vi "OSC UDP Sender.vi"() -> ()   [LabVIEW 2013]
doc: "This example VI shows how to create Open Sound Control (OSC) messages and send them over UDP. This VI is intended to be run with the OSC UDP Receiver example VI."
uses:
  <vilib>/NIOSC/Create Float32 Argument.vi
  <vilib>/NIOSC/Create Double Argument.vi
  <vilib>/NIOSC/Create Boolean Argument.vi
  <vilib>/NIOSC/Create String Argument.vi
  <vilib>/NIOSC/Generate Error.vi
  <vilib>/NIOSC/Pad String.vi
  <vilib>/NIOSC/Check for Valid String Data.vi
  <vilib>/NIOSC/Multiple of 32.vi
  <vilib>/NIOSC/Create Message_Single Arg.vi
  <vilib>/NIOSC/Create Message_Multiple Args.vi
  <vilib>/NIOSC/NI_OSC.lvlib
panel:
  in  "/group4/data":T1
  in  "/group3/bool/*":bool
  in  "/group3/bool/c":bool
  in  "/group3/bool/b":bool
  in  "/group3/bool/a":bool
  in  "//float64//":dbl(slide) scale=-100.0..100.0
  in  "/group2/float64/num_a":dbl
  in  "/group2/float32/num_b":sgl
  in  "//float32//":sgl(slide) scale=-100.0..100.0
  in  "Yslide":sgl(slide) scale=-1.0..1.0
  in  "Zout":sgl(slide) scale=-20.0..10.0
  in  "Broadcast":bool
  in  "Remote Host":string="localhost"
  in  "Remote Port":u16=9000
  in  "Local Port":u16=7000
  in  "stop":bool
  # "Instructions:\n1. Open the receiver VI (OSC UDP Receiver.vi).\n2. Make sure the Remote Port in this VI and the Local Port in the receiver VI are the same.\n3. Run both VIs.\n4. Change the values of the controls on this VI to observe how OSC messages are created.  The indicators on the receiver VI should update."
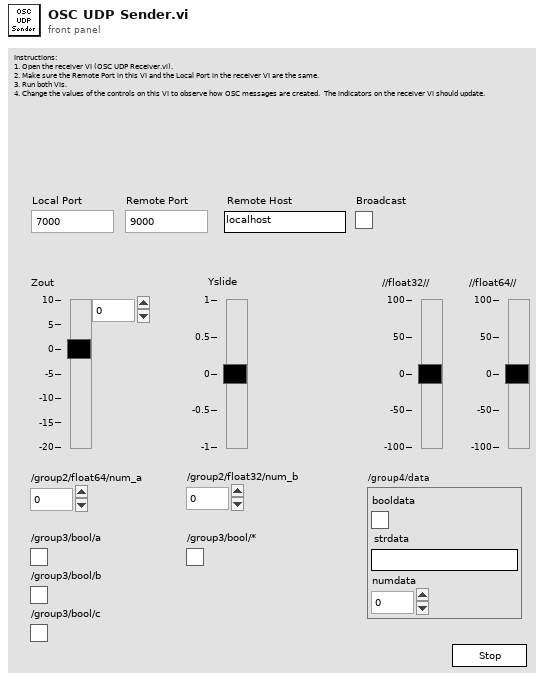
[diagram p1: front panel]
types:
  T1 = cluster{"booldata":bool, "strdata":string, "numdata":dbl}
  T2 = typedef "NI_OSC.lvlib/Argument.ctl" = cluster{"argument":string, "type tag":string}
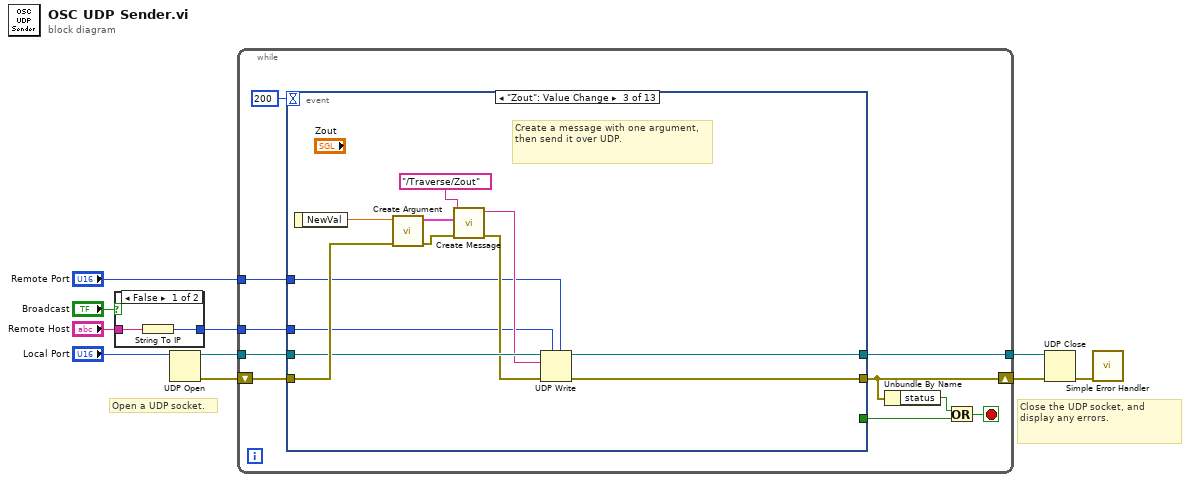
[diagram p0: block diagram]
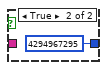
[diagram p2: hidden frame]
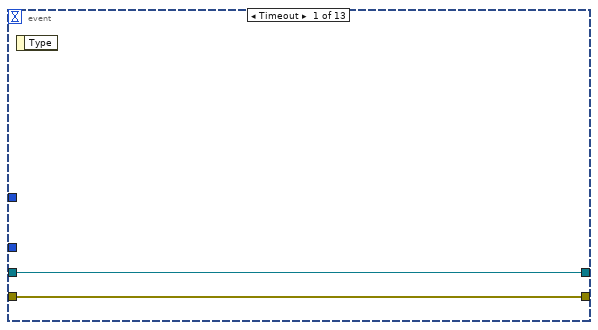
[diagram p3: hidden frame]
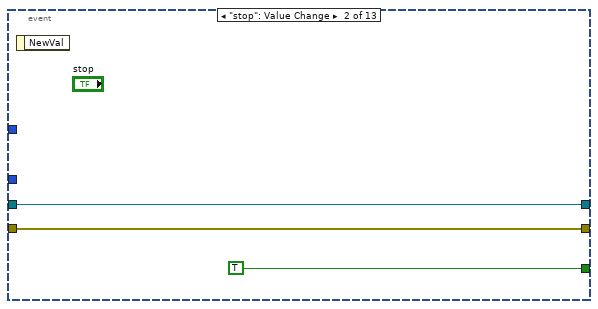
[diagram p4: hidden frame]
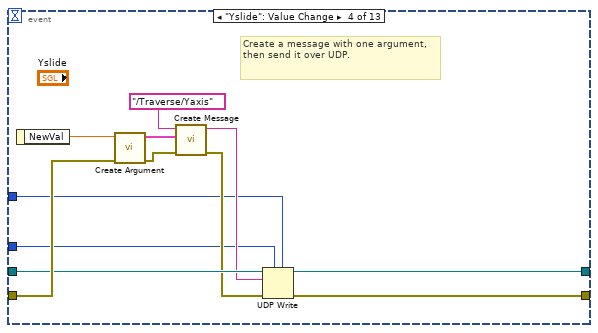
[diagram p5: hidden frame]
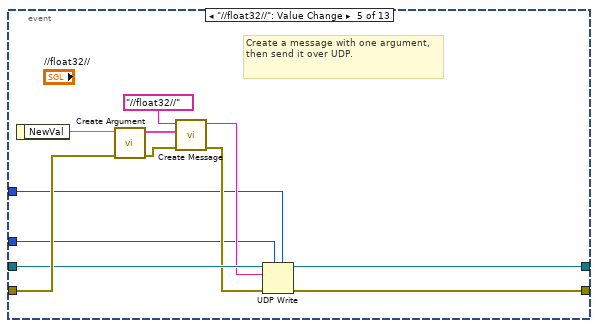
[diagram p6: hidden frame]
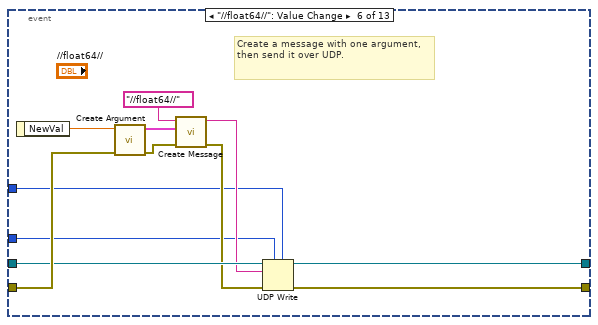
[diagram p7: hidden frame]
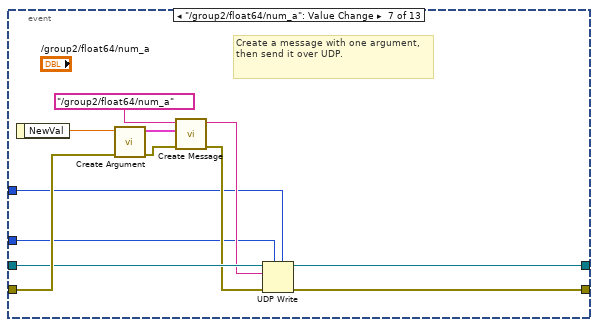
[diagram p8: hidden frame]
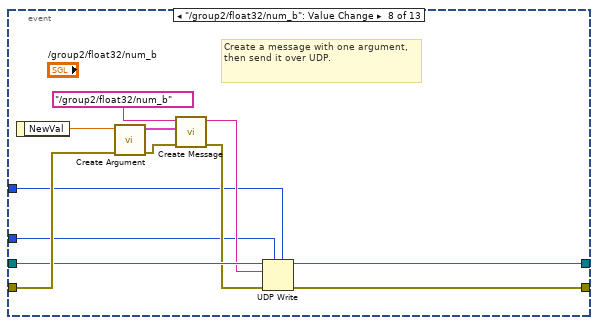
[diagram p9: hidden frame]
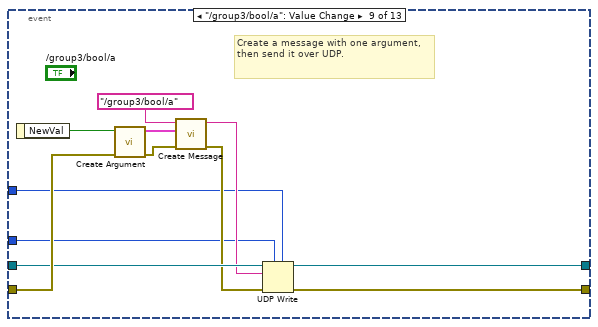
[diagram p10: hidden frame]
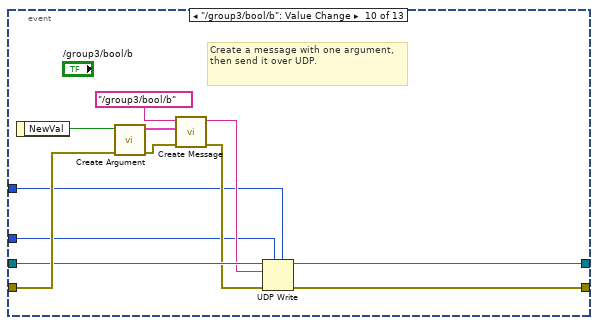
[diagram p11: hidden frame]
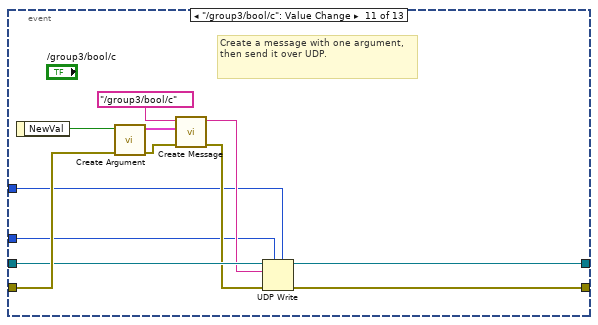
[diagram p12: hidden frame]
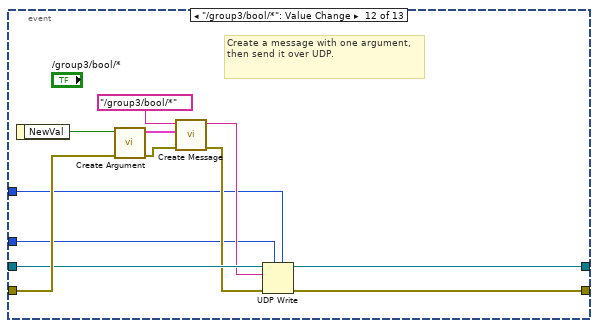
[diagram p13: hidden frame]
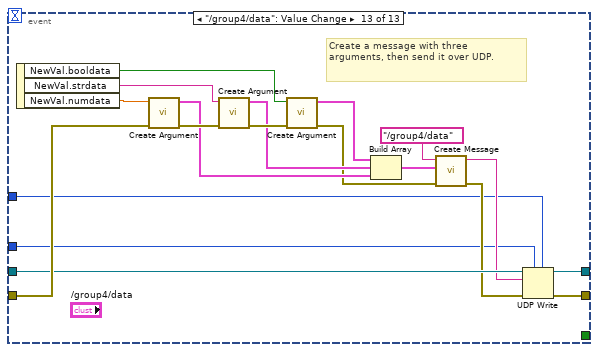
[diagram p14: hidden frame]
diagram:
  # "Close the UDP socket, and display any errors."
  # "Open a UDP socket."
  n1 = case shown="False" "Broadcast" {
    tunnel: "Remote Host" -> [w12 _]
    tunnel: [w11 u32 4294967295] -> w2
    frame False {
      n2 = String To IP(1:w12) -> (0:w11:u32)
    }
    frame True {
    }
  }
  n3 = UDP Open(11:"Local Port") -> (port=w9:refnum<k16>, 0:w8:errorcluster)  [unwired: 4 in, 1 out]
  n4 = while {
    tunnel: w9 -> [w22]
    shift-right: [w17] -> w5
    shift-left: w8 -> [w21]
    tunnel: "Remote Port" -> [w20]
    tunnel: [w19] -> w6
    tunnel: w2 -> [w18]
    stop <- w14 stop-if-true
    n5 = event shown="[2] \"Zout\": Value Change" {
      selector: _ -> [_ _ _ _ _ _ _ _ _ _ _ _ _]
      dyn-events: _ -> [_ _ _ _ _ _ _ _ _ _ _ _ _]
      timeout: 200 -> [_ _ _ _ _ _ _ _ _ _ _ _ _]
      tunnel: [_ TRUE _ _ _ _ _ _ _ _ _ _ _] -> w16
      tunnel: w22 -> [w25 w27 w36 w47 w59 w72 w84 w96 w108 w120 w132 w144 w165]
      tunnel: w21 -> [w24 w26 w37 w48 w60 w73 w85 w97 w109 w121 w133 w145 w166]
      tunnel: w20 -> [_ _ w32 w43 w55 w68 w80 w92 w104 w116 w128 w140 w161]
      tunnel: [w25 w27 w35 w46 w58 w71 w83 w95 w107 w119 w131 w143 w164] -> w19
      tunnel: [w24 w26 w30 w41 w53 w66 w78 w90 w102 w114 w126 w138 w159] -> w17
      tunnel: w18 -> [_ _ w31 w42 w54 w67 w79 w91 w103 w115 w127 w139 w160]
      event Timeout {
        n6 = event-data() -> ()  [unwired: 1 in, 1 out]
      }
      event "stop": Value Change {
        n7 = event-data() -> ()  [unwired: 1 in, 1 out]
      }
      event "Zout": Value Change {
        # "Create a message with one argument, then send it over UDP."
        n8 = event-data() -> ("NewVal"=w29:sgl)  [unwired: 1 in]
        n9 = call-poly <vilib>:"Create Argument.vi"("error in"=w37, "float32 data"=w29) -> ("error out"=w38:errorcluster, "float32 argument"=w40:T2)  [unwired: 8 in]
        n10 = call-poly <vilib>:"Create Message.vi"("error in"=w38, "argument"=w40, "address pattern"="/Traverse/Zout") -> ("error out"=w34:errorcluster, "message"=w33:string)  [unwired: 7 in]
        n11 = UDP Write(address=w31, port or service name=w32, connection ID=w36, data in=w33, 8:w34) -> (error out=w30:errorcluster, 3:w35:refnum<k16>)  [unwired: 1 in]
      }
      event "Yslide": Value Change {
        # "Create a message with one argument, then send it over UDP."
        n12 = event-data() -> ("NewVal"=w52:sgl)  [unwired: 1 in]
        n13 = call-poly <vilib>:"Create Argument.vi"("error in"=w48, "float32 data"=w52) -> ("error out"=w49:errorcluster, "float32 argument"=w51:T2)  [unwired: 8 in]
        n14 = call-poly <vilib>:"Create Message.vi"("error in"=w49, "argument"=w51, "address pattern"="/Traverse/Yaxis") -> ("error out"=w45:errorcluster, "message"=w44:string)  [unwired: 7 in]
        n15 = UDP Write(address=w42, port or service name=w43, connection ID=w47, data in=w44, 8:w45) -> (error out=w41:errorcluster, 3:w46:refnum<k16>)  [unwired: 1 in]
      }
      event "//float32//": Value Change {
        # "Create a message with one argument, then send it over UDP."
        n16 = event-data() -> ("NewVal"=w64:sgl)  [unwired: 1 in]
        n17 = call-poly <vilib>:"Create Argument.vi"("error in"=w60, "float32 data"=w64) -> ("error out"=w61:errorcluster, "float32 argument"=w63:T2)  [unwired: 8 in]
        n18 = call-poly <vilib>:"Create Message.vi"("error in"=w61, "argument"=w63, "address pattern"="//float32//") -> ("error out"=w57:errorcluster, "message"=w56:string)  [unwired: 7 in]
        n19 = UDP Write(address=w54, port or service name=w55, connection ID=w59, data in=w56, 8:w57) -> (error out=w53:errorcluster, 3:w58:refnum<k16>)  [unwired: 1 in]
      }
      event "//float64//": Value Change {
        # "Create a message with one argument, then send it over UDP."
        n20 = event-data() -> ("NewVal"=w65:dbl)  [unwired: 1 in]
        n21 = call-poly <vilib>:"Create Argument.vi"("error in"=w73, "double data"=w65) -> ("error out"=w74:errorcluster, "double argument"=w76:T2)  [unwired: 8 in]
        n22 = call-poly <vilib>:"Create Message.vi"("error in"=w74, "argument"=w76, "address pattern"="//float64//") -> ("error out"=w70:errorcluster, "message"=w69:string)  [unwired: 7 in]
        n23 = UDP Write(address=w67, port or service name=w68, connection ID=w72, data in=w69, 8:w70) -> (error out=w66:errorcluster, 3:w71:refnum<k16>)  [unwired: 1 in]
      }
      event "/group2/float64/num_a": Value Change {
        # "Create a message with one argument, then send it over UDP."
        n24 = event-data() -> ("NewVal"=w77:dbl)  [unwired: 1 in]
        n25 = call-poly <vilib>:"Create Argument.vi"("error in"=w85, "double data"=w77) -> ("error out"=w86:errorcluster, "double argument"=w88:T2)  [unwired: 8 in]
        n26 = call-poly <vilib>:"Create Message.vi"("error in"=w86, "argument"=w88, "address pattern"="/group2/float64/num_a") -> ("error out"=w82:errorcluster, "message"=w81:string)  [unwired: 7 in]
        n27 = UDP Write(address=w79, port or service name=w80, connection ID=w84, data in=w81, 8:w82) -> (error out=w78:errorcluster, 3:w83:refnum<k16>)  [unwired: 1 in]
      }
      event "/group2/float32/num_b": Value Change {
        # "Create a message with one argument, then send it over UDP."
        n28 = event-data() -> ("NewVal"=w89:sgl)  [unwired: 1 in]
        n29 = call-poly <vilib>:"Create Argument.vi"("error in"=w97, "float32 data"=w89) -> ("error out"=w98:errorcluster, "float32 argument"=w100:T2)  [unwired: 8 in]
        n30 = call-poly <vilib>:"Create Message.vi"("error in"=w98, "argument"=w100, "address pattern"="/group2/float32/num_b") -> ("error out"=w94:errorcluster, "message"=w93:string)  [unwired: 7 in]
        n31 = UDP Write(address=w91, port or service name=w92, connection ID=w96, data in=w93, 8:w94) -> (error out=w90:errorcluster, 3:w95:refnum<k16>)  [unwired: 1 in]
      }
      event "/group3/bool/a": Value Change {
        # "Create a message with one argument, then send it over UDP."
        n32 = event-data() -> ("NewVal"=w101:bool)  [unwired: 1 in]
        n33 = call-poly <vilib>:"Create Argument.vi"("error in"=w109, "boolean data"=w101) -> ("error out"=w110:errorcluster, "boolean argument"=w112:T2)  [unwired: 8 in]
        n34 = call-poly <vilib>:"Create Message.vi"("error in"=w110, "argument"=w112, "address pattern"="/group3/bool/a") -> ("error out"=w106:errorcluster, "message"=w105:string)  [unwired: 7 in]
        n35 = UDP Write(address=w103, port or service name=w104, connection ID=w108, data in=w105, 8:w106) -> (error out=w102:errorcluster, 3:w107:refnum<k16>)  [unwired: 1 in]
      }
      event "/group3/bool/b": Value Change {
        # "Create a message with one argument, then send it over UDP."
        n36 = event-data() -> ("NewVal"=w113:bool)  [unwired: 1 in]
        n37 = call-poly <vilib>:"Create Argument.vi"("error in"=w121, "boolean data"=w113) -> ("error out"=w122:errorcluster, "boolean argument"=w124:T2)  [unwired: 8 in]
        n38 = call-poly <vilib>:"Create Message.vi"("error in"=w122, "argument"=w124, "address pattern"="/group3/bool/b") -> ("error out"=w118:errorcluster, "message"=w117:string)  [unwired: 7 in]
        n39 = UDP Write(address=w115, port or service name=w116, connection ID=w120, data in=w117, 8:w118) -> (error out=w114:errorcluster, 3:w119:refnum<k16>)  [unwired: 1 in]
      }
      event "/group3/bool/c": Value Change {
        # "Create a message with one argument, then send it over UDP."
        n40 = event-data() -> ("NewVal"=w125:bool)  [unwired: 1 in]
        n41 = call-poly <vilib>:"Create Argument.vi"("error in"=w133, "boolean data"=w125) -> ("error out"=w134:errorcluster, "boolean argument"=w136:T2)  [unwired: 8 in]
        n42 = call-poly <vilib>:"Create Message.vi"("error in"=w134, "argument"=w136, "address pattern"="/group3/bool/c") -> ("error out"=w130:errorcluster, "message"=w129:string)  [unwired: 7 in]
        n43 = UDP Write(address=w127, port or service name=w128, connection ID=w132, data in=w129, 8:w130) -> (error out=w126:errorcluster, 3:w131:refnum<k16>)  [unwired: 1 in]
      }
      event "/group3/bool/*": Value Change {
        # "Create a message with one argument, then send it over UDP."
        n44 = event-data() -> ("NewVal"=w137:bool)  [unwired: 1 in]
        n45 = call-poly <vilib>:"Create Argument.vi"("error in"=w145, "boolean data"=w137) -> ("error out"=w146:errorcluster, "boolean argument"=w148:T2)  [unwired: 8 in]
        n46 = call-poly <vilib>:"Create Message.vi"("error in"=w146, "argument"=w148, "address pattern"="/group3/bool/*") -> ("error out"=w142:errorcluster, "message"=w141:string)  [unwired: 7 in]
        n47 = UDP Write(address=w139, port or service name=w140, connection ID=w144, data in=w141, 8:w142) -> (error out=w138:errorcluster, 3:w143:refnum<k16>)  [unwired: 1 in]
      }
      event "/group4/data": Value Change {
        # "Create a message with three arguments, then send it over UDP."
        n48 = event-data() -> ("NewVal.booldata"=w155:bool, "NewVal.strdata"=w156:string, "NewVal.numdata"=w158:dbl)  [unwired: 1 in]
        n49 = call-poly <vilib>:"Create Argument.vi"("error in"=w166, "double data"=w158) -> ("error out"=w157:errorcluster, "double argument"=w151:T2)  [unwired: 8 in]
        n50 = call-poly <vilib>:"Create Argument.vi"("error in"=w157, "string data"=w156) -> ("error out"=w154:errorcluster, "string argument"=w152:T2)  [unwired: 8 in]
        n51 = call-poly <vilib>:"Create Argument.vi"("error in"=w154, "boolean data"=w155) -> ("error out"=w149:errorcluster, "boolean argument"=w153:T2)  [unwired: 8 in]
        n52 = Build Array(w153, w152, w151) -> (w150:T2[])
        n53 = call-poly <vilib>:"Create Message.vi"("error in"=w149, "arguments"=w150, "address pattern"="/group4/data") -> ("error out"=w163:errorcluster, "message"=w162:string)  [unwired: 7 in]
        n54 = UDP Write(address=w160, port or service name=w161, connection ID=w165, data in=w162, 8:w163) -> (error out=w159:errorcluster, 3:w164:refnum<k16>)  [unwired: 1 in]
      }
    }
    n55 = Unbundle By Name(w17) -> ("status"=w15:bool)
    n56 = Or(x=w15, y=w16) -> (x .or. y?=w14:bool)
  }
  n57 = UDP Close(connection ID=w6, 8:w5) -> (error out=w1:errorcluster)  [unwired: 1 out]
  n58 = call <vilib>:"Simple Error Handler.vi"("error in (no error)"=w1) -> ()  [unwired: 4 in, 5 out]
